vi "PM5020 SCPI Example.vi"() -> ()   [LabVIEW 2013]
uses:
  <vilib>/ErrorRing/Error Ring.xnode
  <vilib>/Utility/error.llb/Error Cluster From Error Code.vi
panel:
  in  "stop":bool
  out "ARR LEN":i32
  out "rate":dbl format="%#.2f"
  out "count":i32
  out "time":u32
  out "error out":errorcluster
  in  "Tab Control":T1(tab)
  out "Chart":dbl(graph)
  in  "Scope Mode Array Length":i32=100
  out "Scope Mode Array [timestamp(us), power(W), power(W)]":cluster{u32, sgl, sgl}[](array[cluster])
  in  "Burst Mode Array Length":i32=100
  out "Burst Mode Array [timestamp(us), power(W), power(W)]":cluster{u32, sgl, sgl}[](array[cluster])
  out "Product Info":string
  # "Average Sampling Rate (Samples/s)"
  # "(range is 1 to 100)"
  # "I/O ports are 5 V TTL tolerant. The start of measurement is triggered on the rising edge of the TTL signal. In this example, connect Pin5 (TRIG) and Pin6 (GND) of the rear DIGITAL I/O port to the external TTL signal source."
  # "(range is 1 to 100)"
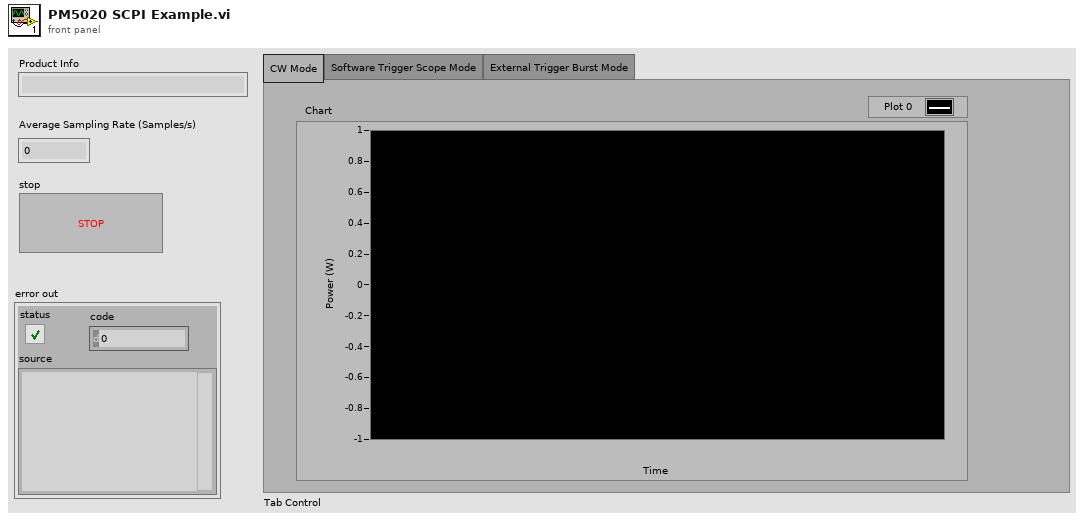
[diagram p1: front panel]
types:
  T1 = enum32{"CW Mode", "Software Trigger Scope Mode", "External Trigger Burst Mode"}
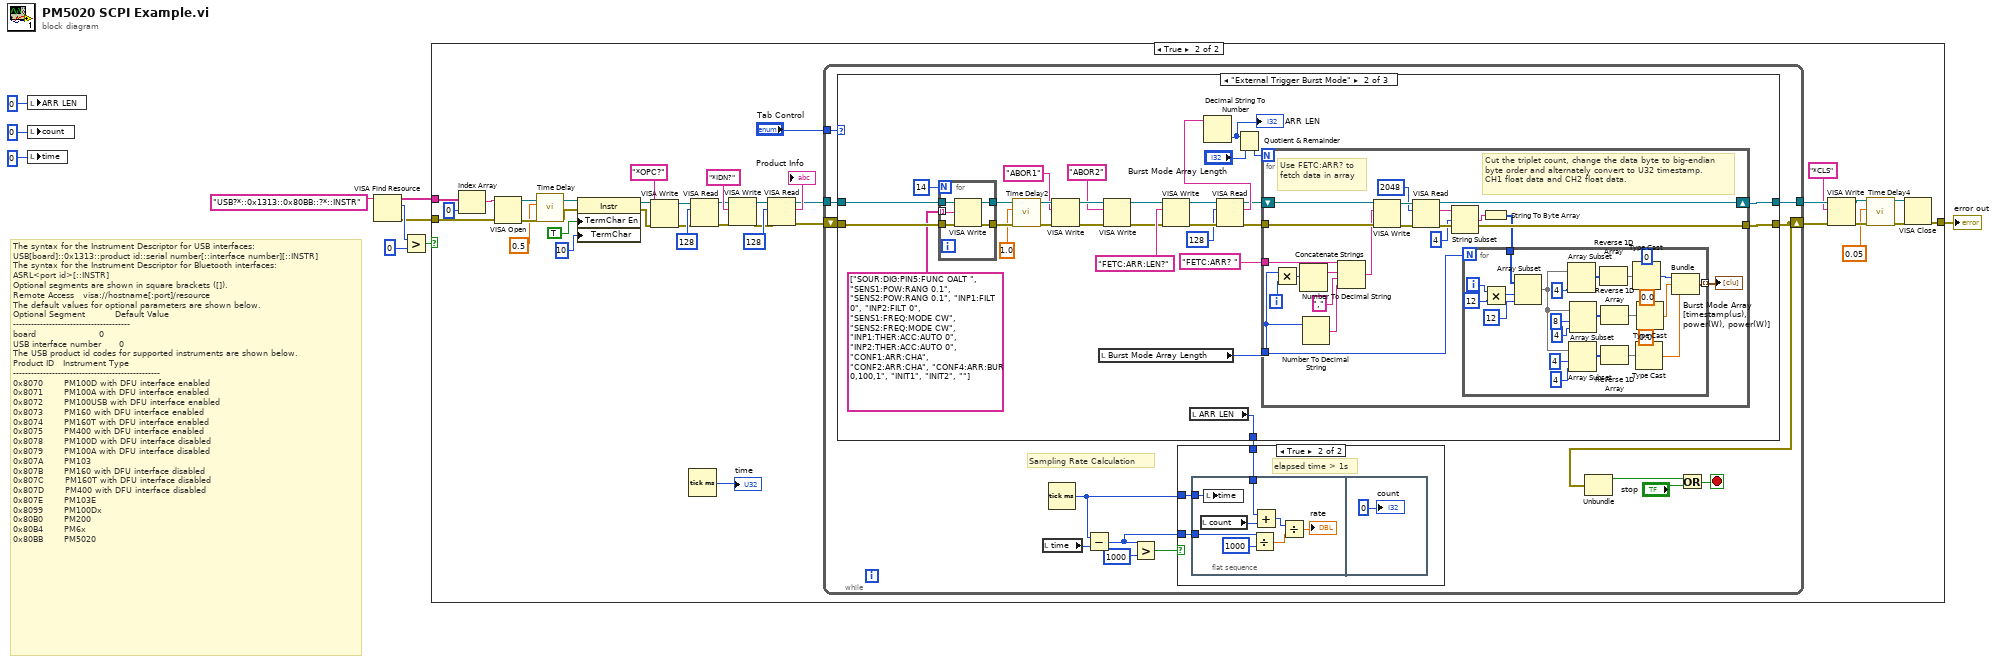
[diagram p0: block diagram]
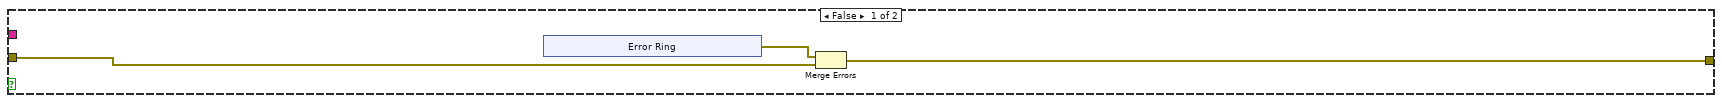
[diagram p2: hidden frame]
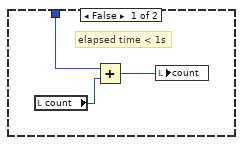
[diagram p3: hidden frame]
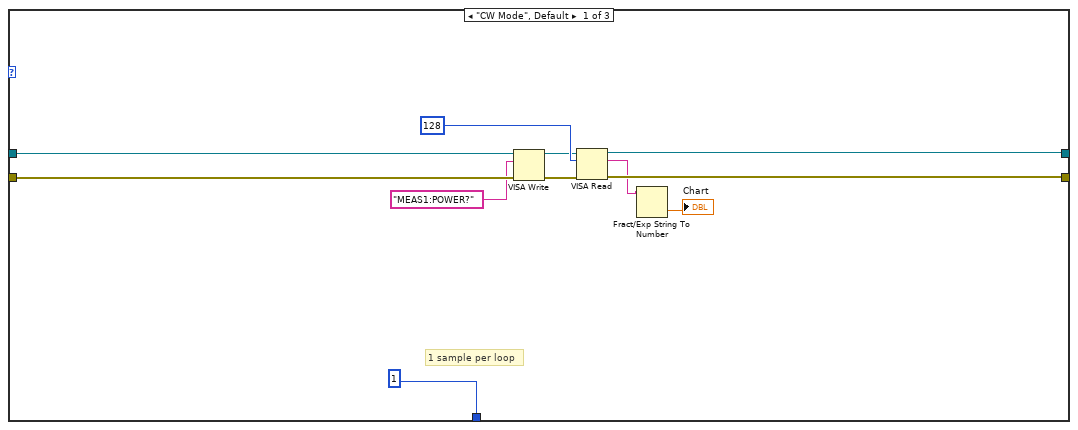
[diagram p4: hidden frame]
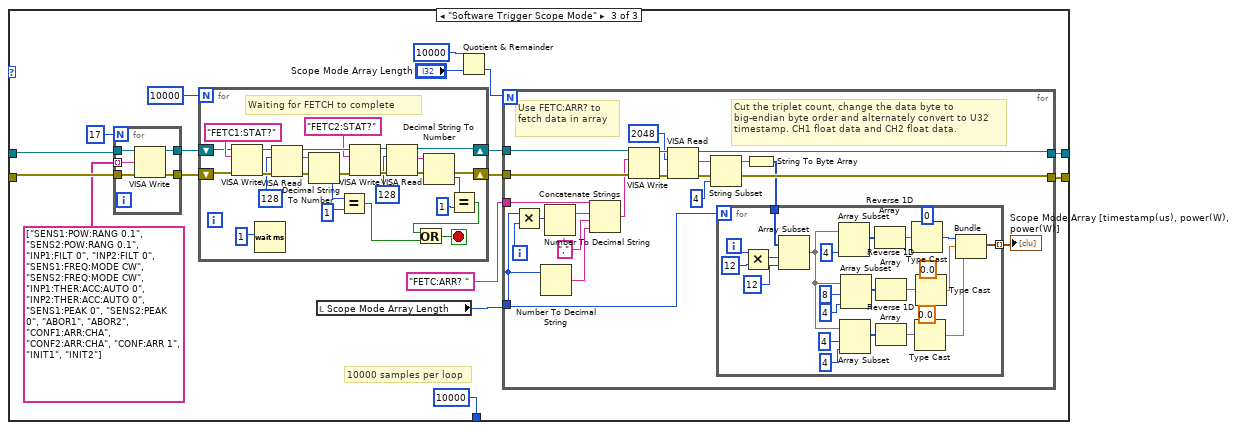
[diagram p5: hidden frame]
diagram:
  # "The syntax for the Instrument Descriptor for USB interfaces:\nUSB[board]::0x1313::product id::serial number[::interface number][::INSTR]\nThe syntax for the Instrument Descriptor for Bluetooth interfaces:\nASRL<port id>[::INSTR]\nOptional segments are shown in square brackets ([]).\nRemote Access   visa://hostname[:port]/resource\nThe default values for optional parameters are shown below.\nOptional Segment          Default Value\n---------------------------------------\nboard                     0\nUSB interface number      0\nThe USB product id codes for supported instruments are shown below.\nProduct ID   Instrument Type\n-------------------------------------------------\n0x8070       PM100D with DFU interface enabled\n0x8071       PM100A with DFU interface enabled\n0x8072       PM100USB with DFU interface enabled\n0x8073       PM160 with DFU interface enabled\n0x8074       PM160T with DFU interface enabled\n0x8075       PM400 with DFU interface enabled\n0x8078       PM100D with DFU interface disabled\n0x8079       PM100A with DFU interface disabled\n0x807A       PM103\n0x807B       PM160 with DFU interface disabled\n0x807C       PM160T with DFU interface disabled\n0x807D       PM400 with DFU interface disabled\n0x807E       PM103E\n0x8099       PM100Dx\n0x80B0       PM200\n0x80B4       PM6x\n0x80BB       PM5020"
  n1 = local write "ARR LEN"(0 ("ARR LEN")) -> ()
  n2 = local write "count"(0 ("loopCount")) -> ()
  n3 = local write "time"(u32 0 ("time")) -> ()
  n4 = VISA Find Resource(11:"USB?*::0x1313::0x80BB::?*::INSTR" ("expression (\"?*\")")) -> (0:w4:errorcluster, 2:w9:u32, 3:w6:string[])  [unwired: 2 in]
  n5 = Greater?(x=w9, y=u32 0) -> (0:w7:bool)
  n6 = case shown="True" w7 {
    tunnel: w6 -> [_ w53]
    tunnel: [w13 w26] -> w5
    tunnel: w4 -> [w12 w38]
    frame False {
      n7 = xnode "Error Ring"() -> ("error out"=w11:errorcluster)
      n8 = Merge Errors(w11, w12) -> (w13:errorcluster)
    }
    frame True {
      n9 = Index Array(array=w53, index=0) -> (element=w39:string)
      n10 = VISA Open(error in (no error)=w38, VISA resource name=w39) -> (VISA resource name=w45:refnum<visa-resource-name>, error out=w48:errorcluster)  [unwired: 3 in]
      n11 = call "Time Delay"("error in (no error)"=w48, "Delay Time (s)"=0.5) -> ("error out"=w46:errorcluster)  [unwired: 9 in]
      n12 = property class="Instr"(reference=w45, error in=w46, "TermChar En"=TRUE ("Message Based Settings:Termination Character Enable"), "TermChar"=u8 10 ("Message Based Settings:Termination Character")) -> (reference out=w22:refnum<visa-resource-name>, error out=w21:errorcluster)
      n13 = VISA Write(VISA resource name=w22, write buffer="*OPC?", error in (no error)=w21) -> (VISA resource name out=w34:refnum<visa-resource-name>, error out=w19:errorcluster)  [unwired: 1 out]
      n14 = Tick Count (ms)() -> (millisecond timer value=→"time":u32)
      n15 = VISA Read(VISA resource name=w34, byte count=u32 128, error in (no error)=w19) -> (VISA resource name out=w33:refnum<visa-resource-name>, error out=w36:errorcluster)  [unwired: 2 out]
      n16 = VISA Write(VISA resource name=w33, write buffer="*IDN?", error in (no error)=w36) -> (VISA resource name out=w50:refnum<visa-resource-name>, error out=w25:errorcluster)  [unwired: 1 out]
      n17 = VISA Read(VISA resource name=w50, byte count=u32 128, error in (no error)=w25) -> (VISA resource name out=w42:refnum<visa-resource-name>, read buffer=→"Product Info":string, error out=w41:errorcluster)  [unwired: 1 out]
      n18 = while {
        tunnel: [w67] -> w31
        tunnel: w42 -> [w66]
        tunnel: "Tab Control" -> [w64]
        shift-right: [w56] -> w32
        shift-left: w41 -> [w65]
        stop <- w54 stop-if-true
        # "Sampling Rate Calculation"
        n19 = case shown="\"External Trigger Burst Mode\"" w64 {
          tunnel: [w90 w120 w186] -> w67
          tunnel: w66 -> [w92 w121 w187]
          tunnel: [w89 w122 w188] -> w56
          tunnel: w65 -> [w91 w119 w185]
          tunnel: [1 w118 10000 ("x")] -> w61
          frame "CW Mode", Default {
            # "1 sample per loop"
            n20 = VISA Write(VISA resource name=w92, write buffer="MEAS1:POWER?", error in (no error)=w91) -> (VISA resource name out=w84:refnum<visa-resource-name>, error out=w83:errorcluster)  [unwired: 1 out]
            n21 = VISA Read(VISA resource name=w84, byte count=u32 128, error in (no error)=w83) -> (VISA resource name out=w90:refnum<visa-resource-name>, read buffer=w87:string, error out=w89:errorcluster)  [unwired: 1 out]
            n22 = Fract/Exp String To Number(string=w87) -> (number=→"Chart":dbl)  [unwired: 3 in, 1 out]
          }
          frame "External Trigger Burst Mode" {
            n23 = for {
              N: 14 -> [_]
              tunnel: string[] ["SOUR:DIG:PIN5:FUNC OALT ", "SENS1:POW:RANG 0.1", "SENS2:POW:RANG 0.1", "INP1:FILT 0", "INP2:FILT 0", "SENS1:FREQ:MODE CW", "SENS2:FREQ:MODE CW", "INP1:THER:ACC:AUTO 0", "INP2:THER:ACC:AUTO 0", "CONF1:ARR:CHA", "CONF2:ARR:CHA", "CONF4:ARR:BUR 0,100,1", "INIT1", "INIT2", ""] -> [w169] mode=indexing
              tunnel: w119 -> [w171]
              tunnel: w121 -> [w170]
              tunnel: [w168] -> w115
              tunnel: [w167] -> w112
              n24 = VISA Write(VISA resource name=w170, write buffer=w169, error in (no error)=w171) -> (VISA resource name out=w167:refnum<visa-resource-name>, error out=w168:errorcluster)  [unwired: 1 out]
            }
            n25 = call "Time Delay2"("error in (no error)"=w115, "Delay Time (s)"=1.0) -> ("error out"=w113:errorcluster)  [unwired: 9 in]
            n26 = VISA Write(VISA resource name=w112, write buffer="ABOR1", error in (no error)=w113) -> (VISA resource name out=w97:refnum<visa-resource-name>, error out=w98:errorcluster)  [unwired: 1 out]
            n27 = local read "Burst Mode Array Length"() -> (w99:i32)
            n28 = VISA Write(VISA resource name=w97, write buffer="ABOR2", error in (no error)=w98) -> (VISA resource name out=w96:refnum<visa-resource-name>, error out=w95:errorcluster)  [unwired: 1 out]
            n29 = VISA Write(VISA resource name=w96, write buffer="FETC:ARR:LEN?", error in (no error)=w95) -> (VISA resource name out=w108:refnum<visa-resource-name>, error out=w109:errorcluster)  [unwired: 1 out]
            n30 = local read "ARR LEN"() -> (w118:i32)
            n31 = VISA Read(VISA resource name=w108, byte count=u32 128, error in (no error)=w109) -> (VISA resource name out=w104:refnum<visa-resource-name>, read buffer=w106:string, error out=w105:errorcluster)  [unwired: 1 out]
            n32 = Decimal String To Number(string=w106) -> (number=w102:i32)  [unwired: 2 in, 1 out]
            "ARR LEN" <- w102
            n33 = Quotient & Remainder(x=w102, y="Burst Mode Array Length") -> (floor(x/y)=w100:i32)  [unwired: 1 out]
            n34 = for {
              N: w100 -> [_]
              tunnel: w105 -> [w142]
              tunnel: "FETC:ARR? " ("write buffer") -> [w133]
              tunnel: [w128] -> w122
              tunnel: w99 -> [w125]
              shift-right: [w129] -> w120
              shift-left: w104 -> [w140]
              i -> [w131]
              # "Cut the triplet count, change the data byte to big-endian byte order and alternately convert to U32 timestamp. CH1 float data and CH2 float data."
              # "Use FETC:ARR? to fetch data in array"
              n35 = Multiply(x=w125, y=w131) -> (x*y=w135:i32)
              n36 = Number To Decimal String(number=w135) -> (decimal integer string=w137:string)  [unwired: 1 in]
              n37 = Number To Decimal String(number=w125) -> (decimal integer string=w134:string)  [unwired: 1 in]
              n38 = Concatenate Strings(w133, w137, "," ("string"), w134) -> (w132:string)
              n39 = VISA Write(VISA resource name=w140, write buffer=w132, error in (no error)=w142) -> (VISA resource name out=w139:refnum<visa-resource-name>, error out=w141:errorcluster)  [unwired: 1 out]
              n40 = VISA Read(VISA resource name=w139, byte count=u32 2048, error in (no error)=w141) -> (VISA resource name out=w129:refnum<visa-resource-name>, read buffer=w130:string, error out=w128:errorcluster)  [unwired: 1 out]
              n41 = String Subset(string=w130, offset (0)=4) -> (substring=w127:string)  [unwired: 1 in]
              n42 = String To Byte Array(string=w127) -> (unsigned byte array=w126:u8[])
              n43 = for {
                N: w125 -> [_]
                tunnel: w126 -> [w145]
                tunnel: [w144] -> w124 mode=indexing
                i -> [w146]
                n44 = Multiply(x=w146, y=12) -> (x*y=w166:i32)
                n45 = Array Subset(array=w145, index=w166, length=12) -> (w150:u8[])
                n46 = Array Subset(array=w150, length=4) -> (w157:u8[])  [unwired: 1 in]
                n47 = Array Subset(array=w150, index=4, length=4) -> (w152:u8[])
                n48 = Array Subset(array=w150, index=8, length=4) -> (w155:u8[])
                n49 = Reverse 1D Array(array=w157) -> (reversed array=w156:u8[])
                n50 = Reverse 1D Array(array=w155) -> (reversed array=w154:u8[])
                n51 = Reverse 1D Array(array=w152) -> (reversed array=w151:u8[])
                n52 = Type Cast(type=u32 0, x=w156) -> (*(type *) &x=w159:u32)
                n53 = Type Cast(type=sgl 0.0, x=w151) -> (*(type *) &x=w147:sgl)
                n54 = Type Cast(type=sgl 0.0, x=w154) -> (*(type *) &x=w158:sgl)
                n55 = Bundle(w159, w158, w147) -> (w144:cluster{u32, sgl, sgl})  [unwired: 1 in]
              }
              "Burst Mode Array [timestamp(us), power(W), power(W)]" <- w124
            }
          }
          frame "Software Trigger Scope Mode" {
            # "10000 samples per loop"
            n56 = for {
              N: 17 -> [_]
              tunnel: w185 -> [w261]
              tunnel: w187 -> [w260]
              tunnel: [w259] -> w178
              tunnel: [w258] -> w182
              tunnel: string[] ["SENS1:POW:RANG 0.1", "SENS2:POW:RANG 0.1", "INP1:FILT 0", "INP2:FILT 0", "SENS1:FREQ:MODE CW", "SENS2:FREQ:MODE CW", "INP1:THER:ACC:AUTO 0", "INP2:THER:ACC:AUTO 0", "SENS1:PEAK 0", "SENS2:PEAK 0", "ABOR1", "ABOR2", "CONF1:ARR:CHA", "CONF2:ARR:CHA", "CONF:ARR 1", "INIT1", "INIT2"] -> [w257] mode=indexing
              n57 = VISA Write(VISA resource name=w260, write buffer=w257, error in (no error)=w261) -> (VISA resource name out=w258:refnum<visa-resource-name>, error out=w259:errorcluster)  [unwired: 1 out]
            }
            n58 = for {
              N: 10000 -> [_]
              shift-right: [w202] -> w180
              shift-left: w182 -> [w205]
              shift-right: [w199] -> w179
              shift-left: w178 -> [w208]
              stop <- w189 stop-if-true
              # "Waiting for FETCH to complete"
              n59 = VISA Write(VISA resource name=w205, write buffer="FETC1:STAT?", error in (no error)=w208) -> (VISA resource name out=w211:refnum<visa-resource-name>, error out=w207:errorcluster)  [unwired: 1 out]
              n60 = Wait (ms)(milliseconds to wait=u32 1) -> ()  [unwired: 1 out]
              n61 = VISA Read(VISA resource name=w211, byte count=u32 128, error in (no error)=w207) -> (VISA resource name out=w204:refnum<visa-resource-name>, read buffer=w210:string, error out=w201:errorcluster)  [unwired: 1 out]
              n62 = Decimal String To Number(string=w210) -> (number=w194:i32)  [unwired: 2 in, 1 out]
              n63 = Equal?(x=w194, y=1) -> (x = y?=w190:bool)
              n64 = VISA Write(VISA resource name=w204, write buffer="FETC2:STAT?", error in (no error)=w201) -> (VISA resource name out=w203:refnum<visa-resource-name>, error out=w200:errorcluster)  [unwired: 1 out]
              n65 = VISA Read(VISA resource name=w203, byte count=u32 128, error in (no error)=w200) -> (VISA resource name out=w202:refnum<visa-resource-name>, read buffer=w192:string, error out=w199:errorcluster)  [unwired: 1 out]
              n66 = Decimal String To Number(string=w192) -> (number=w196:i32)  [unwired: 2 in, 1 out]
              n67 = Equal?(x=w196, y=1) -> (x = y?=w191:bool)
              n68 = Or(x=w191, y=w190) -> (x .or. y?=w189:bool)
            }
            n69 = local read "Scope Mode Array Length"() -> (w173:i32)
            n70 = Quotient & Remainder(x=10000, y="Scope Mode Array Length") -> (floor(x/y)=w176:i32)  [unwired: 1 out]
            n71 = for {
              N: w176 -> [_]
              tunnel: w179 -> [w232]
              tunnel: w180 -> [w230]
              tunnel: "FETC:ARR? " ("write buffer") -> [w228]
              tunnel: [w224] -> w186
              tunnel: w173 -> [w215]
              tunnel: [w218] -> w188
              i -> [w221]
              # "Cut the triplet count, change the data byte to big-endian byte order and alternately convert to U32 timestamp. CH1 float data and CH2 float data."
              # "Use FETC:ARR? to fetch data in array"
              n72 = Multiply(x=w215, y=w221) -> (x*y=w222:i32)
              n73 = Number To Decimal String(number=w215) -> (decimal integer string=w220:string)  [unwired: 1 in]
              n74 = Number To Decimal String(number=w222) -> (decimal integer string=w227:string)  [unwired: 1 in]
              n75 = Concatenate Strings(w228, w227, "," ("string"), w220) -> (w226:string)
              n76 = VISA Write(VISA resource name=w230, write buffer=w226, error in (no error)=w232) -> (VISA resource name out=w229:refnum<visa-resource-name>, error out=w231:errorcluster)  [unwired: 1 out]
              n77 = VISA Read(VISA resource name=w229, byte count=u32 2048, error in (no error)=w231) -> (VISA resource name out=w224:refnum<visa-resource-name>, read buffer=w217:string, error out=w218:errorcluster)  [unwired: 1 out]
              n78 = String Subset(string=w217, offset (0)=4) -> (substring=w219:string)  [unwired: 1 in]
              n79 = String To Byte Array(string=w219) -> (unsigned byte array=w216:u8[])
              n80 = for {
                N: w215 -> [_]
                tunnel: w216 -> [w256]
                tunnel: [w245] -> w213 mode=indexing
                i -> [w254]
                n81 = Multiply(x=w254, y=12) -> (x*y=w255:i32)
                n82 = Array Subset(array=w256, index=w255, length=12) -> (w237:u8[])
                n83 = Array Subset(array=w237, length=4) -> (w244:u8[])  [unwired: 1 in]
                n84 = Array Subset(array=w237, index=4, length=4) -> (w239:u8[])
                n85 = Array Subset(array=w237, index=8, length=4) -> (w242:u8[])
                n86 = Reverse 1D Array(array=w244) -> (reversed array=w243:u8[])
                n87 = Reverse 1D Array(array=w242) -> (reversed array=w241:u8[])
                n88 = Reverse 1D Array(array=w239) -> (reversed array=w238:u8[])
                n89 = Type Cast(type=u32 0, x=w243) -> (*(type *) &x=w247:u32)
                n90 = Type Cast(type=sgl 0.0, x=w238) -> (*(type *) &x=w234:sgl)
                n91 = Type Cast(type=sgl 0.0, x=w241) -> (*(type *) &x=w246:sgl)
                n92 = Bundle(w247, w246, w234) -> (w245:cluster{u32, sgl, sgl})  [unwired: 1 in]
              }
              "Scope Mode Array [timestamp(us), power(W), power(W)]" <- w213
            }
          }
        }
        n93 = local read "time"() -> (w60:u32)
        n94 = Tick Count (ms)() -> (millisecond timer value=w62:u32)
        n95 = Subtract(x=w62, y=w60) -> (x-y=w59:u32)
        n96 = Greater?(x=w59, y=u32 1000) -> (0:w55:bool)
        n97 = case shown="True" w55 {
          tunnel: w62 -> [_ w73]
          tunnel: w61 -> [w69 w71]
          tunnel: w59 -> [_ w72]
          frame False {
            # "elapsed time < 1s"
            n98 = local read "count"() -> (w70:i32)
            n99 = Add(x=w69, y=w70) -> (x+y=w68:i32)
            n100 = local write "count"(w68) -> ()
          }
          frame True {
            # "elapsed time > 1s"
            n101 = flat-sequence {
              tunnel: w73 -> [w81]
              tunnel: w72 -> [w78]
              tunnel: w71 -> [w74]
              frame #0 {
                n102 = local read "count"() -> (w75:i32)
                n103 = local write "time"(w81) -> ()
                n104 = Divide(x=w78, y=u32 1000) -> (x/y=w79:dbl)
                n105 = Add(x=w74, y=w75) -> (x+y=w76:i32)
                n106 = Divide(x=w76, y=w79) -> (x/y=→"rate":dbl)
              }
              frame #1 {
                "count" <- 0 ("count")
              }
            }
          }
        }
        n107 = Unbundle(w56) -> ("status"=w57:bool)  [unwired: 2 out]
        n108 = Or(x=w57, y="stop") -> (x .or. y?=w54:bool)
      }
      n109 = VISA Write(VISA resource name=w31, write buffer="*CLS", error in (no error)=w32) -> (VISA resource name out=w30:refnum<visa-resource-name>, error out=w28:errorcluster)  [unwired: 1 out]
      n110 = call "Time Delay4"("error in (no error)"=w28, "Delay Time (s)"=0.05) -> ("error out"=w27:errorcluster)  [unwired: 9 in]
      n111 = VISA Close(VISA resource name=w30, error in (no error)=w27) -> (error out=w26:errorcluster)
    }
  }
  "error out" <- w5
